vi "move.vi"(10 "Vitesse":dbl, 11 "Angle":dbl) -> ()   [LabVIEW 2015]
uses:
  Variable globale.vi
  <userlib>/ICNC/ICNC2.lvlib
panel:
  in  "Numeric":i32=1
  in  "Deceleration":i32
  in  "Acceleration":i32
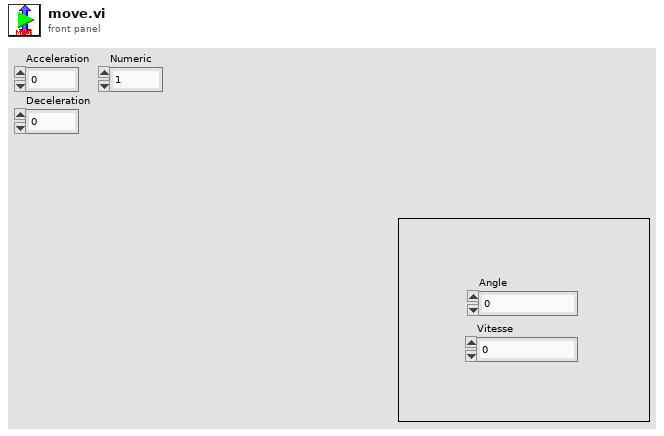
[diagram p1: front panel]
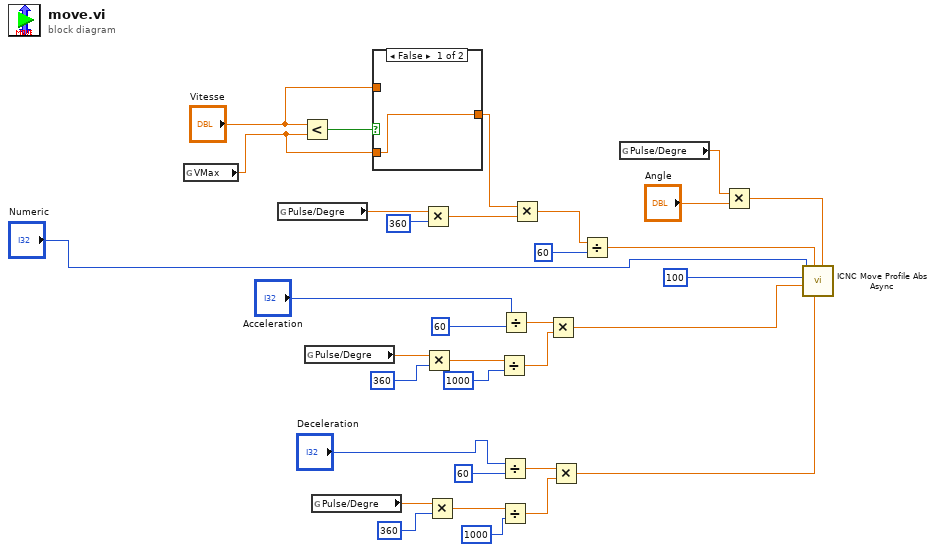
[diagram p0: block diagram]
diagram:
  n1 = global read "Variable globale.vi" "VMax"() -> (w13:dbl)
  n2 = global read "Variable globale.vi" "Pulse/Degre"() -> (w22:dbl)
  n3 = Less?(x="Vitesse", y=w13) -> (x < y?=w15:bool)
  n4 = global read "Variable globale.vi" "Pulse/Degre"() -> (w31:dbl)
  n5 = global read "Variable globale.vi" "Pulse/Degre"() -> (w25:dbl)
  n6 = case shown="False" w15 {
    tunnel: "Vitesse" -> [_ w35]
    tunnel: w13 -> [w34 _]
    tunnel: [w34 w35] -> w9
    frame False {
    }
    frame True {
    }
  }
  n7 = Multiply(x=w22, y=360) -> (x*y=w10:dbl)
  n8 = Multiply(x=w31, y=360) -> (x*y=w12:dbl)
  n9 = Multiply(x=w25, y=360) -> (x*y=w11:dbl)
  n10 = Divide(x=w12, y=1000) -> (x/y=w32:dbl)
  n11 = Divide(x="Deceleration", y=60) -> (x/y=w27:dbl)
  n12 = Divide(x=w11, y=1000) -> (x/y=w26:dbl)
  n13 = Divide(x="Acceleration", y=60) -> (x/y=w19:dbl)
  n14 = Multiply(x=w9, y=w10) -> (x*y=w18:dbl)
  n15 = Multiply(x=w19, y=w32) -> (x*y=w5:dbl)
  n16 = Multiply(x=w27, y=w26) -> (x*y=w4:dbl)
  n17 = Divide(x=w18, y=60) -> (x/y=w7:dbl)
  n18 = global read "Variable globale.vi" "Pulse/Degre"() -> (w17:dbl)
  n19 = Multiply(x=w17, y="Angle") -> (x*y=w8:dbl)
  n20 = call <userlib>:"ICNC Move Profile Abs Async.vi"("Position"=w8, "Decel"=w4, "Speed"=w7, "Accel"=w5, "FStartStop"=100, "Axe"="Numeric") -> ()  [unwired: 4 in, 2 out]
